vi "get runtime class name.vi"(8 "error in":errorcluster, 11 "asynchronous execution module configuration In":refnum<class "asynchronous execution module configuration.lvclass">) -> (0 "error out":errorcluster, 2 "class name":string, 3 "asynchronous execution module configuration Out":refnum<class "asynchronous execution module configuration.lvclass">)   [LabVIEW 2013, in "asynchronous execution module configuration.lvclass"]
doc: "Provides an interface for determining the component runtime class associated with this component configuration. This class name can then be used to dynamically load or locate the runtime class for initialization purposes."
uses:
  asynchronous execution module configuration.lvclass
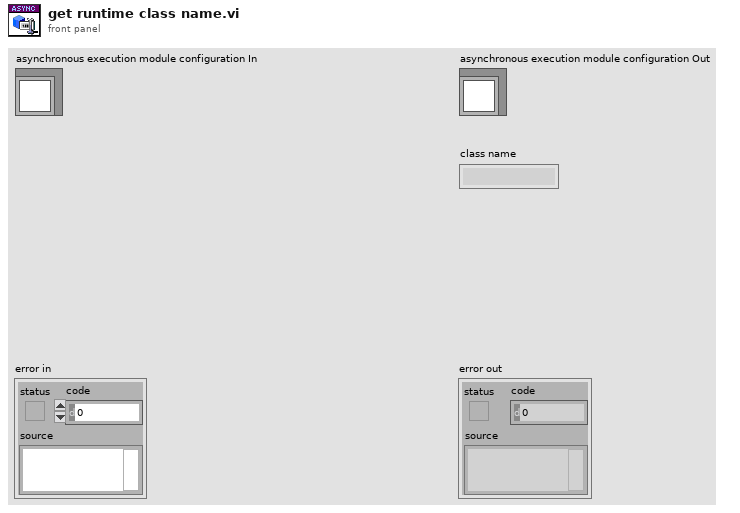
[diagram p1: front panel]
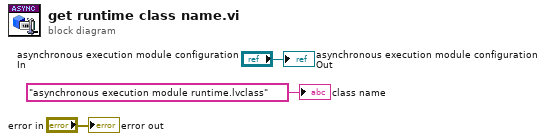
[diagram p0: block diagram]
diagram:
  "error out" <- "error in"
  "asynchronous execution module configuration Out" <- "asynchronous execution module configuration In"
  "class name" <- "asynchronous execution module runtime.lvclass" ("class name")
